vi "Time delay (SubVI).vi"(7 "Ton":dbl, 8 "input":dbl) -> (1 "Output":dbl)   [LabVIEW 2016]
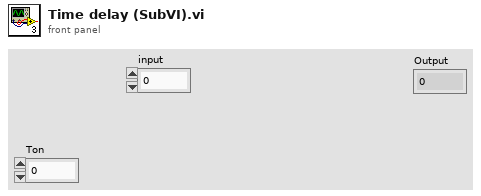
[diagram p1: front panel]
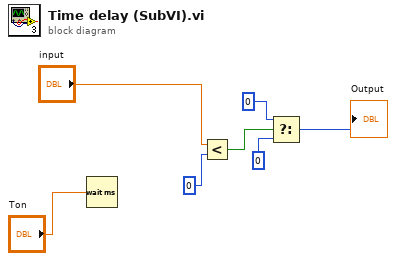
[diagram p0: block diagram]
diagram:
  n1 = Wait (ms)(milliseconds to wait="Ton") -> ()  [unwired: 1 out]
  n2 = Less?(x="input", y=0) -> (x < y?=w5:bool)
  n3 = Select(t=0, s=w5, f=0) -> (s? t:f=→"Output":i32)
